vi "Autonomous Mode Bool.vi"   [LabVIEW 2016]
uses:
  Globale Variable/Globale Variable.vi
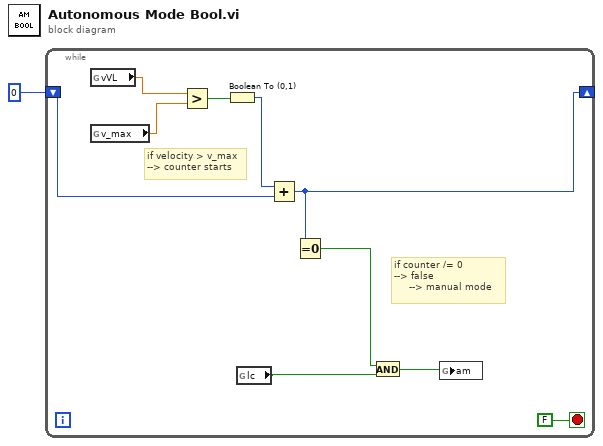
[diagram p0: block diagram]
diagram:
  n1 = while {
    shift-right: [w3] -> _
    shift-left: i16 0 -> [w7]
    stop <- FALSE stop-if-true
    # "if counter /= 0\n--> false \n     --> manual mode"
    # "if velocity > v_max\n--> counter starts"
    n2 = global read "Globale Variable.vi" "vVL"() -> (w11:dbl)
    n3 = global read "Globale Variable.vi" "v_max"() -> (w10:dbl)
    n4 = Greater?(x=w11, y=w10) -> (0:w9:bool)
    n5 = Boolean To (0,1)(Boolean=w9) -> (0, 1=w8:i16)
    n6 = global read "Globale Variable.vi" "lc"() -> (w2:bool)
    n7 = Add(x=w8, y=w7) -> (x+y=w3:i16)
    n8 = Equal To 0?(x=w3) -> (x = 0?=w6:bool)
    n9 = And(x=w6, y=w2) -> (x .and. y?=w5:bool)
    n10 = global write "Globale Variable.vi" "am"(w5) -> ()
  }
